vi "test_read-nmea-data2.vi"() -> ()   [LabVIEW 2019] (continued)
\t\n15:09:12.53\tF9P\t$GLGSV,2,2,08,77,01,327,,84,21,121,11,85,70,063,25,86,35,329,,1*72\n\t\n15:09:12.55\tF9P\t$GLGSV,2,1,08,69,13,031,18,70,73,042,,71,50,204,21,72,03,209,,3*79\n\t\n15:09:12.57\tF9P\t$GLGSV,2,2,08,77,01,327,,84,21,121,18,85,70,063,22,86,35,329,,3*7E\n\t\n15:09:12.59\tF9P\t$GAGSV,2,1,08,02,09,298,09,04,65,120,25,09,30,193,24,11,70,356,26,7*7E\n\t\n15:09:12.61\tF9P\t$GAGSV,2,2,08,12,41,101,23,19,27,046,13,25,10,250,,36,25,307,18,7*7F\n\t\n15:09:12.63\tF9P\t$GAGSV,2,1,08,02,09,298,,04,65,120,28,09,30,193,23,11,70,356,23,2*7D\n\t\n15:09:12.65\tF9P\t$GAGSV,2,2,08,12,41,101,18,19,27,046,,25,10,250,,36,25,307,23,2*78\n\t\n15:09:12.67\tF9P\t$GBGSV,1,1,03,11,51,130,24,14,86,148,24,33,59,218,31,1*40\n\t\n15:09:12.69\tF9P\t$GBGSV,1,1,04,08,,,22,11,51,130,22,14,86,148,26,33,59,218,,3*4B\n\t\n15:09:12.71\tF9P\t$GNGLL,3723.60695,N,12656.91212,E,060914.00,A,A*7B\n\t\n15:09:12.73\tF9P\t\t\n15:09:12.75\tF9P\t\t\n15:09:12.77\tF9P\t\t\n15:09:12.79\tF9P\t\t\n15:09:12.81\tF9P\t\t\n15:09:12.83\tF9P\t\t\n15:09:12.85\tF9P\t\t\n15:09:12.87\tF9P\t\t\n15:09:12.89\tF9P\t\t\n15:09:12.91\tF9P\t\t\n15:09:12.93\tF9P\t\t\n15:09:12.95\tF9P\t\t\n15:09:12.97\tF9P\t\t\n15:09:12.99\tF9P\t\t\n15:09:13.01\tF9P\t\t\n15:09:13.03\tF9P\t\t\n15:09:13.05\tF9P\t\t\n15:09:13.07\tF9P\t\t\n15:09:13.09\tF9P\t\t\n15:09:13.11\tF9P\t\t\n15:09:13.13\tF9P\t\t\n15:09:13.15\tF9P\t\t\n15:09:13.17\tF9P\t\t\n15:09:13.19\tF9P\t\t\n15:09:13.21\tF9P\t\t\n15:09:13.23\tF9P\t\t\n15:09:13.25\tF9P\t$GNRMC,060915.00,A,3723.60643,N,12656.91138,E,3.237,235.26,250720,,,A,V*00\n\t\n15:09:13.27\tF9P\t$GNVTG,235.26,T,,M,3.237,N,5.996,K,A*25\n\t\n15:09:13.30\tF9P\t$GNGGA,060915.00,3723.60643,N,12656.91138,E,1,12,0.73,59.2,M,18.5,M,,*7A\n\t\n15:09:13.32\tF9P\t$GNGSA,A,3,12,06,19,05,17,09,04,02,,,,,1.28,0.73,1.05,1*0B\n\t\n15:09:13.34\tF9P\t$GNGSA,A,3,85,71,84,,,,,,,,,,1.28,0.73,1.05,2*0E\n\t\n15:09:13.36\tF9P\t$GNGSA,A,3,36,19,11,04,09,12,,,,,,,1.28,0.73,1.05,3*0B\n\t\n15:09:13.38\tF9P\t$GNGSA,A,3,14,11,33,,,,,,,,,,1.28,0.73,1.05,4*0A\n\t\n15:09:13.40\tF9P\t$GPGSV,3,1,09,02,54,318,22,04,19,044,19,05,36,246,32,06,65,046,30,1*67\n\t\n15:09:13.42\tF9P\t$GPGSV,3,2,09,09,45,075,33,12,24,278,26,17,35,153,24,19,54,156,34,1*67\n\t\n15:09:13.44\tF9P\t$GPGSV,3,3,09,25,12,308,,1*52\n\t\n15:09:13.46\tF9P\t$GPGSV,3,1,09,02,54,318,,04,19,044,13,05,36,246,17,06,65,046,25,6*69\n\t\n15:09:13.48\tF9P\t$GPGSV,3,2,09,09,45,075,20,12,24,278,18,17,35,153,16,19,54,156,,6*69\n\t\n15:09:13.50\tF9P\t$GPGSV,3,3,09,25,12,308,,6*55\n\t\n15:09:13.52\tF9P\t$GLGSV,2,1,08,69,13,031,,70,73,042,,71,50,204,26,72,03,209,,1*75\n\t\n15:09:13.54\tF9P\t$GLGSV,2,2,08,77,01,327,,84,21,121,09,85,70,063,25,86,35,329,,1*7B\n\t\n15:09:13.56\tF9P\t$GLGSV,2,1,08,69,13,031,16,70,73,042,,71,50,204,22,72,03,209,,3*74\n\t\n15:09:13.58\tF9P\t$GLGSV,2,2,08,77,01,327,,84,21,121,17,85,70,063,21,86,35,329,,3*72\n\t\n15:09:13.60\tF9P\t$GAGSV,2,1,08,02,09,298,11,04,65,120,26,09,30,193,22,11,70,356,27,7*73\n\t\n15:09:13.62\tF9P\t$GAGSV,2,2,08,12,41,101,34,19,27,046,13,25,10,250,,36,25,307,17,7*76\n\t\n15:09:13.64\tF9P\t$GAGSV,2,1,08,02,09,298,,04,65,120,27,09,30,193,24,11,70,356,22,2*74\n\t\n15:09:13.66\tF9P\t$GAGSV,2,2,08,12,41,101,19,19,27,046,,25,10,250,,36,25,307,21,2*7B\n\t\n15:09:13.68\tF9P\t$GBGSV,1,1,03,11,51,130,24,14,86,148,26,33,59,218,31,1*42\n\t\n15:09:13.70\tF9P\t$GBGSV,1,1,04,08,,,23,11,51,130,23,14,86,148,25,33,59,218,,3*48\n\t\n15:09:13.72\tF9P\t$GNGLL,3723.60643,N,12656.91138,E,060915.00,A,A*7A\n\t\n15:09:13.74\tF9P\t\t\n15:09:13.76\tF9P\t\t\n15:09:13.78\tF9P\t\t\n15:09:13.80\tF9P\t\t\n15:09:13.82\tF9P\t\t\n15:09:13.84\tF9P\t\t\n15:09:13.86\tF9P\t\t\n15:09:13.88\tF9P\t\t\n15:09:13.90\tF9P\t\t\n15:09:13.92\tF9P\t\t\n15:09:13.94\tF9P\t\t\n15:09:13.96\tF9P\t\t\n15:09:13.98\tF9P\t\t\n15:09:14.00\tF9P\t\t\n15:09:14.02\tF9P\t\t\n15:09:14.04\tF9P\t\t\n15:09:14.06\tF9P\t\t\n15:09:14.08\tF9P\t\t\n15:09:14.10\tF9P\t\t\n15:09:14.12\tF9P\t\t\n15:09:14.14\tF9P\t\t\n15:09:14.16\tF9P\t\t\n15:09:14.18\tF9P\t\t\n15:09:14.20\tF9P\t\t\n15:09:14.22\tF9P\t\t\n15:09:14.24\tF9P\t\t\n15:09:14.26\tF9P\t$GNRMC,060916.00,A,3723.60597,N,12656.91090,E,1.962,233.87,250720,,,A,V*0E\n\t\n15:09:14.28\tF9P\t$GNVTG,233.87,T,,M,1.962,N,3.634,K,A*20\n\t\n15:09:14.30\tF9P\t$GNGGA,060916.00,3723.60597,N,12656.91090,E,1,12,0.73,59.3,M,18.5,M,,*71\n\t\n15:09:14.32\tF9P\t$GNGSA,A,3,12,06,19,05,17,09,04,02,,,,,1.28,0.73,1.05,1*0B\n\t\n15:09:14.34\tF9P\t$GNGSA,A,3,85,71,84,,,,,,,,,,1.28,0.73,1.05,2*0E\n\t\n15:09:14.36\tF9P\t$GNGSA,A,3,36,19,11,04,09,12,,,,,,,1.28,0.73,1.05,3*0B\n\t\n15:09:14.38\tF9P\t$GNGSA,A,3,14,11,33,,,,,,,,,,1.28,0.73,1.05,4*0A\n\t\n15:09:14.40\tF9P\t$GPGSV,3,1,09,02,54,318,23,04,19,044,19,05,36,246,26,06,65,046,33,1*60\n\t\n15:09:14.42\tF9P\t$GPGSV,3,2,09,09,45,075,29,12,24,278,31,17,34,153,25,19,54,156,31,1*6F\n\t\n15:09:14.44\tF9P\t$GPGSV,3,3,09,25,12,308,,1*52\n\t\n15:09:14.46\tF9P\t$GPGSV,3,1,09,02,54,318,,04,19,044,09,05,36,246,18,06,65,046,23,6*6B\n\t\n15:09:14.48\tF9P\t$GPGSV,3,2,09,09,45,075,22,12,24,278,18,17,34,153,16,19,54,156,,6*6A\n\t\n15:09:14.50\tF9P\t$GPGSV,3,3,09,25,12,308,,6*55\n\t\n15:09:14.52\tF9P\t$GLGSV,2,1,08,69,13,031,,70,73,042,,71,50,204,26,72,03,209,,1*75\n\t\n15:09:14.54\tF9P\t$GLGSV,2,2,08,77,01,327,,84,21,121,09,85,70,063,24,86,35,329,,1*7A\n\t\n15:09:14.56\tF9P\t$GLGSV,2,1,08,69,13,031,18,70,73,042,,71,50,204,21,72,03,209,,3*79\n\t\n15:09:14.58\tF9P\t$GLGSV,2,2,08,77,01,327,,84,21,121,17,85,70,063,21,86,35,329,,3*72\n\t\n15:09:14.60\tF9P\t$GAGSV,2,1,08,02,09,298,07,04,65,120,25,09,30,193,20,11,70,356,24,7*76\n\t\n15:09:14.62\tF9P\t$GAGSV,2,2,08,12,41,101,25,19,27,046,13,25,10,250,,36,25,307,19,7*78\n\t\n15:09:14.64\tF9P\t$GAGSV,2,1,08,02,09,298,,04,65,120,28,09,30,193,21,11,70,356,20,2*7C\n\t\n15:09:14.66\tF9P\t$GAGSV,2,2,08,12,41,101,19,19,27,046,,25,10,250,,36,25,307,27,2*7D\n\t\n15:09:14.68\tF9P\t$GBGSV,1,1,03,11,51,130,23,14,86,148,26,33,59,218,27,1*42\n\t\n15:09:14.70\tF9P\t$GBGSV,1,1,04,08,,,23,11,51,130,24,14,86,148,26,33,59,218,,3*4C\n\t\n15:09:14.72\tF9P\t$GNGLL,3723.60597,N,12656.91090,E,060916.00,A,A*70\n\t\n15:09:14.74\tF9P\t\t\n15:09:14.76\tF9P\t\t\n15:09:14.78\tF9P\t\t\n15:09:14.80\tF9P\t\t\n15:09:14.82\tF9P\t\t\n15:09:14.84\tF9P\t\t\n15:09:14.86\tF9P\t\t\n15:09:14.88\tF9P\t\t\n15:09:14.90\tF9P\t\t\n15:09:14.92\tF9P\t\t\n15:09:14.94\tF9P\t\t\n15:09:14.96\tF9P\t\t\n15:09:14.98\tF9P\t\t\n15:09:15.00\tF9P\t\t\n15:09:15.02\tF9P\t\t\n15:09:15.04\tF9P\t\t\n15:09:15.06\tF9P\t\t\n15:09:15.08\tF9P\t\t\n15:09:15.10\tF9P\t\t\n15:09:15.12\tF9P\t\t\n15:09:15.14\tF9P\t\t\n15:09:15.16\tF9P\t\t\n15:09:15.18\tF9P\t\t\n15:09:15.20\tF9P\t\t\n15:09:15.22\tF9P\t\t\n15:09:15.24\tF9P\t\t\n15:09:15.26\tF9P\t$GNRMC,060917.00,A,3723.60562,N,12656.91048,E,2.165,237.78,250720,,,A,V*08\n\t\n15:09:15.28\tF9P\t$GNVTG,237.78,T,,M,2.165,N,4.009,K,A*27\n\t\n15:09:15.30\tF9P\t$GNGGA,060917.00,3723.60562,N,12656.91048,E,1,12,0.67,59.3,M,18.5,M,,*7A\n\t\n15:09:15.32\tF9P\t$GNGSA,A,3,12,06,19,05,17,09,04,02,,,,,1.21,0.67,1.02,1*00\n\t\n15:09:15.34\tF9P\t$GNGSA,A,3,85,71,84,,,,,,,,,,1.21,0.67,1.02,2*05\n\t\n15:09:15.36\tF9P\t$GNGSA,A,3,36,19,11,04,09,12,,,,,,,1.21,0.67,1.02,3*00\n\t\n15:09:15.38\tF9P\t$GNGSA,A,3,14,11,33,,,,,,,,,,1.21,0.67,1.02,4*01\n\t\n15:09:15.40\tF9P\t$GPGSV,3,1,09,02,54,318,23,04,19,044,19,05,36,246,26,06,65,046,23,1*61\n\t\n15:09:15.42\tF9P\t$GPGSV,3,2,09,09,45,075,34,12,24,278,31,17,34,153,24,19,54,156,25,1*67\n\t\n15:09:15.44\tF9P\t$GPGSV,3,3,09,25,12,308,,1*52\n\t\n15:09:15.46\tF9P\t$GPGSV,3,1,09,02,54,318,,04,19,044,12,05,36,246,17,06,65,046,22,6*6F\n\t\n15:09:15.48\tF9P\t$GPGSV,3,2,09,09,45,075,22,12,24,278,18,17,34,153,15,19,54,156,,6*69\n\t\n15:09:15.50\tF9P\t$GPGSV,3,3,09,25,12,308,,6*55\n\t\n15:09:15.52\tF9P\t$GLGSV,2,1,08,69,13,031,,70,73,042,,71,50,204,31,72,03,209,,1*73\n\t\n15:09:15.54\tF9P\t$GLGSV,2,2,08,77,01,327,,84,21,121,10,85,70,063,31,86,35,329,,1*76\n\t\n15:09:15.56\tF9P\t$GLGSV,2,1,08,69,13,031,23,70,73,042,,71,50,204,22,72,03,209,,3*72\n\t\n15:09:15.58\tF9P\t$GLGSV,2,2,08,77,01,327,,84,21,121,18,85,70,063,20,86,35,329,,3*7C\n\t\n15:09:15.60\tF9P\t$GAGSV,2,1,08,02,09,298,11,04,65,120,25,09,30,193,22,11,70,356,23,7*74\n\t\n15:09:15.62\tF9P\t$GAGSV,2,2,08,12,41,101,24,19,27,046,13,25,10,250,,36,25,307,19,7*79\n\t\n15:09:15.64\tF9P\t$GAGSV,2,1,08,02,09,298,,04,65,120,32,09,30,193,20,11,70,356,20,2*76\n\t\n15:09:15.66\tF9P\t$GAGSV,2,2,08,12,41,101,19,19,27,046,,25,10,250,,36,25,307,28,2*72\n\t\n15:09:15.68\tF9P\t$GBGSV,1,1,03,11,51,130,23,14,86,148,26,33,59,218,27,1*42\n\t\n15:09:15.70\tF9P\t$GBGSV,1,1,04,08,,,22,11,51,130,21,14,86,148,26,33,59,218,,3*48\n\t\n15:09:15.72\tF9P\t$GNGLL,3723.60562,N,12656.91048,E,060917.00,A,A*7E\n\t\n15:09:15.74\tF9P\t\t\n15:09:15.76\tF9P\t\t\n15:09:15.78\tF9P\t\t\n15:09:15.80\tF9P\t\t\n15:09:15.82\tF9P\t\t\n15:09:15.84\tF9P\t\t\n15:09:15.86\tF9P\t\t\n15:09:15.88\tF9P\t\t\n15:09:15.90\tF9P\t\t\n15:09:15.92\tF9P\t\t\n15:09:15.94\tF9P\t\t\n15:09:15.96\tF9P\t\t\n15:09:15.98\tF9P\t\t\n15:09:16.00\tF9P\t\t\n15:09:16.02\tF9P\t\t\n15:09:16.04\tF9P\t\t\n15:09:16.06\tF9P\t\t\n15:09:16.08\tF9P\t\t\n15:09:16.10\tF9P\t\t\n15:09:16.12\tF9P\t\t\n15:09:16.14\tF9P\t\t\n15:09:16.16\tF9P\t\t\n15:09:16.18\tF9P\t\t\n15:09:16.20\tF9P\t\t\n15:09:16.22\tF9P\t\t\n15:09:16.24\tF9P\t\t\n15:09:16.26\tF9P\t$GNRMC,060918.00,A,3723.60529,N,12656.90999,E,2.086,239.76,250720,,,A,V*00\n\t\n15:09:16.28\tF9P\t$GNVTG,239.76,T,,M,2.086,N,3.863,K,A*28\n\t\n15:09:16.30\tF9P\t$GNGGA,060918.00,3723.60529,N,12656.90999,E,1,12,0.66,59.4,M,18.5,M,,*78\n\t\n15:09:16.32\tF9P\t$GNGSA,A,3,12,06,19,05,17,09,04,02,,,,,1.21,0.66,1.02,1*01\n\t\n15:09:16.34\tF9P\t$GNGSA,A,3,85,71,84,,,,,,,,,,1.21,0.66,1.02,2*04\n\t\n15:09:16.36\tF9P\t$GNGSA,A,3,36,19,11,04,09,12,,,,,,,1.21,0.66,1.02,3*01\n\t\n15:09:16.38\tF9P\t$GNGSA,A,3,14,11,33,,,,,,,,,,1.21,0.66,1.02,4*00\n\t\n15:09:16.40\tF9P\t$GPGSV,3,1,09,02,54,318,22,04,19,044,19,05,36,246,26,06,65,046,25,1*66\n\t\n15:09:16.42\tF9P\t$GPGSV,3,2,09,09,45,075,34,12,24,278,24,17,34,153,25,19,53,156,25,1*65\n\t\n15:09:16.44\tF9P\t$GPGSV,3,3,09,25,12,308,,1*52\n\t\n15:09:16.46\tF9P\t$GPGSV,3,1,09,02,54,318,,04,19,044,15,05,36,246,17,06,65,046,24,6*6E\n\t\n15:09:16.48\tF9P\t$GPGSV,3,2,09,09,45,075,22,12,24,278,17,17,34,153,13,19,53,156,,6*67\n\t\n15:09:16.50\tF9P\t$GPGSV,3,3,09,25,12,308,,6*55\n\t\n15:09:16.52\tF9P\t$GLGSV,2,1,08,69,13,031,,70,73,042,,71,50,204,34,72,03,209,,1*76\n\t\n15:09:16.54\tF9P\t$GLGSV,2,2,08,77,01,327,,84,21,121,12,85,70,063,24,86,35,329,,1*70\n\t\n15:09:16.56\tF9P\t$GLGSV,2,1,08,69,13,031,22,70,73,042,,71,50,204,24,72,03,209,,3*75\n\t\n15:09:16.58\tF9P\t$GLGSV,2,2,08,77,01,327,,84,21,121,17,85,70,063,20,86,35,329,,3*73\n\t\n15:09:16.60\tF9P\t$GAGSV,2,1,08,02,09,298,12,04,65,120,25,09,30,193,23,11,70,356,23,7*76\n\t\n15:09:16.62\tF9P\t$GAGSV,2,2,08,12,41,101,25,19,27,046,15,25,10,250,,36,25,307,19,7*7E\n\t\n15:09:16.64\tF9P\t$GAGSV,2,1,08,02,09,298,,04,65,120,27,09,30,193,20,11,70,356,22,2*70\n\t\n15:09:16.66\tF9P\t$GAGSV,2,2,08,12,41,101,17,19,27,046,,25,10,250,,36,25,307,27,2*73\n\t\n15:09:16.68\tF9P\t$GBGSV,1,1,03,11,51,130,22,14,86,148,25,33,59,218,26,1*41\n\t\n15:09:16.70\tF9P\t$GBGSV,1,1,04,08,,,21,11,51,130,22,14,86,148,26,33,59,218,,3*48\n\t\n15:09:16.72\tF9P\t$GNGLL,3723.60529,N,12656.90999,E,060918.00,A,A*7A\n\t\n15:09:16.74\tF9P\t\t\n15:09:16.76\tF9P\t\t\n15:09:16.78\tF9P\t\t\n15:09:16.80\tF9P\t\t\n15:09:16.82\tF9P\t\t\n15:09:16.84\tF9P\t\t\n15:09:16.86\tF9P\t\t\n15:09:16.88\tF9P\t\t\n15:09:16.90\tF9P\t\t\n15:09:16.92\tF9P\t\t\n15:09:16.94\tF9P\t\t\n15:09:16.96\tF9P\t\t\n15:09:16.98\tF9P\t\t\n15:09:17.00\tF9P\t\t\n15:09:17.02\tF9P\t\t\n15:09:17.04\tF9P\t\t\n15:09:17.06\tF9P\t\t\n15:09:17.08\tF9P\t\t\n15:09:17.10\tF9P\t\t\n15:09:17.12\tF9P\t\t\n15:09:17.14\tF9P\t\t\n15:09:17.16\tF9P\t\t\n15:09:17.18\tF9P\t\t\n15:09:17.20\tF9P\t\t\n15:09:17.22\tF9P\t\t\n15:09:17.24\tF9P\t$GNRMC,060919.00,A,3723.60505,N,12656.90947,E,1.416,,250720,,,A,\t\n15:09:17.26\tF9P\tV*15\n\t\n15:09:17.28\tF9P\t$GNVTG,,T,,M,1.416,N,2.622,K,A*3B\n\t\n15:09:17.30\tF9P\t$GNGGA,060919.00,3723.60505,N,12656.90947,E,1,12,0.76,59.2,M,18.5,M,,*73\n\t\n15:09:17.32\tF9P\t$GNGSA,A,3,12,06,19,05,17,09,04,02,,,,,1.33,0.76,1.09,1*08\n\t\n15:09:17.34\tF9P\t$GNGSA,A,3,85,71,84,,,,,,,,,,1.33,0.76,1.09,2*0D\n\t\n15:09:17.36\tF9P\t$GNGSA,A,3,36,19,11,04,09,12,,,,,,,1.33,0.76,1.09,3*08\n\t\n15:09:17.38\tF9P\t$GNGSA,A,3,14,11,33,,,,,,,,,,1.33,0.76,1.09,4*09\n\t\n15:09:17.40\tF9P\t$GPGSV,3,1,09,02,54,318,22,04,19,044,19,05,36,246,32,06,65,046,31,1*66\n\t\n15:09:17.42\tF9P\t$GPGSV,3,2,09,09,45,075,29,12,24,278,30,17,34,153,25,19,53,156,25,1*6C\n\t\n15:09:17.44\tF9P\t$GPGSV,3,3,09,25,12,308,,1*52\n\t\n15:09:17.46\tF9P\t$GPGSV,3,1,09,02,54,318,,04,19,044,15,05,36,246,18,06,65,046,25,6*60\n\t\n15:09:17.48\tF9P\t$GPGSV,3,2,09,09,45,075,19,12,24,278,18,17,34,153,13,19,53,156,,6*60\n\t\n15:09:17.50\tF9P\t$GPGSV,3,3,09,25,12,308,,6*55\n\t\n15:09:17.52\tF9P\t$GLGSV,2,1,08,69,13,031,,70,73,042,,71,50,204,30,72,03,209,,1*72\n\t\n15:09:17.54\tF9P\t$GLGSV,2,2,08,77,01,327,,84,21,121,13,85,70,063,30,86,35,329,,1*74\n\t\n15:09:17.56\tF9P\t$GLGSV,2,1,08,69,13,031,20,70,73,042,,71,50,204,23,72,03,209,,3*70\n\t\n15:09:17.58\tF9P\t$GLGSV,2,2,08,77,01,327,,84,21,121,16,85,70,063,21,86,35,329,,3*73\n\t\n15:09:17.60\tF9P\t$GAGSV,2,1,08,02,09,298,12,04,65,120,23,09,30,193,30,11,70,356,23,7*72\n\t\n15:09:17.62\tF9P\t$GAGSV,2,2,08,12,41,101,23,19,27,046,09,25,10,250,,36,25,307,18,7*74\n\t\n15:09:17.64\tF9P\t$GAGSV,2,1,08,02,09,298,,04,65,120,25,09,30,193,20,11,70,356,20,2*70\n\t\n15:09:17.66\tF9P\t$GAGSV,2,2,08,12,41,101,18,19,27,046,,25,10,250,,36,25,307,25,2*7E\n\t\n15:09:17.68\tF9P\t$GBGSV,1,1,03,11,51,130,22,14,86,148,25,33,59,218,26,1*41\n\t\n15:09:17.70\tF9P\t$GBGSV,1,1,04,08,,,23,11,51,130,22,14,86,148,25,33,59,218,,3*49\n\t\n15:09:17.72\tF9P\t$GNGLL,3723.60505,N,12656.90947,E,060919.00,A,A*76\n\t\n15:09:17.74\tF9P\t\t\n15:09:17.76\tF9P\t\t\n15:09:17.78\tF9P\t\t\n15:09:17.80\tF9P\t\t\n15:09:17.82\tF9P\t\t\n15:09:17.84\tF9P\t\t\n15:09:17.86\tF9P\t\t\n15:09:17.88\tF9P\t\t\n15:09:17.90\tF9P\t\t\n15:09:17.92\tF9P\t\t\n15:09:17.94\tF9P\t\t\n15:09:17.96\tF9P\t\t\n15:09:17.98\tF9P\t\t\n15:09:18.00\tF9P\t\t\n15:09:18.02\tF9P\t\t\n15:09:18.04\tF9P\t\t\n15:09:18.06\tF9P\t\t\n15:09:18.08\tF9P\t\t\n15:09:18.10\tF9P\t\t\n15:09:18.12\tF9P\t\t\n15:09:18.14\tF9P\t\t\n15:09:18.16\tF9P\t\t\n15:09:18.18\tF9P\t\t\n15:09:18.20\tF9P\t\t\n15:09:18.22\tF9P\t\t\n15:09:18.24\tF9P\t$GNRMC,060920.00,A,3723.60487,N,12656.90892,E,1.791,,250720,,,A,V*11\n\t\n15:09:18.26\tF9P\t$GNVTG,,T,,M,1.791,N,3.317,K,A*35\n\t\n15:09:18.28\tF9P\t$GNGGA,060920.00,3723.60487,N,12656.90892,E,1,12,0.73,59.7,M,18.5,M,,*7B\n\t\n15:09:18.30\tF9P\t$GNGSA,A,3,12,06,19,05,17,09,04,02,,,,,1.28,0.73,1.05,1*0B\n\t\n15:09:18.32\tF9P\t$GNGSA,A,3,85,71,84,,,,,,,,,,1.28,0.73,1.05,2*0E\n\t\n15:09:18.34\tF9P\t$GNGSA,A,3,36,19,11,04,09,12,,,,,,,1.28,0.73,1.05,3*0B\n\t\n15:09:18.36\tF9P\t$GNGSA,A,3,14,11,33,,,,,,,,,,1.28,0.73,1.05,4*0A\n\t\n15:09:18.38\tF9P\t$GPGSV,3,1,09,02,54,318,21,04,19,044,20,05,36,246,18,06,65,046,31,1*67\n\t\n15:09:18.40\tF9P\t$GPGSV,3,2,09,09,45,075,30,12,24,278,29,17,34,153,24,19,53,156,24,1*6C\n\t\n15:09:18.42\tF9P\t$GPGSV,3,3,09,25,12,308,,1*52\n\t\n15:09:18.44\tF9P\t$GPGSV,3,1,09,02,54,318,,04,19,044,16,05,36,246,18,06,65,046,24,6*62\n\t\n15:09:18.46\tF9P\t$GPGSV,3,2,09,09,45,075,18,12,24,278,18,17,34,153,11,19,53,156,,6*63\n\t\n15:09:18.48\tF9P\t$GPGSV,3,3,09,25,12,308,,6*55\n\t\n15:09:18.50\tF9P\t$GLGSV,2,1,08,69,13,031,,70,73,042,,71,50,204,29,72,03,209,,1*7A\n\t\n15:09:18.52\tF9P\t$GLGSV,2,2,08,77,01,327,,84,21,121,09,85,70,063,23,86,35,329,,1*7D\n\t\n15:09:18.54\tF9P\t$GLGSV,2,1,08,69,13,031,16,70,73,042,,71,50,204,22,72,03,209,,3*74\n\t\n15:09:18.56\tF9P\t$GLGSV,2,2,08,77,01,327,,84,21,121,16,85,70,063,21,86,35,329,,3*73\n\t\n15:09:18.58\tF9P\t$GAGSV,2,1,08,02,09,298,10,04,65,120,23,09,30,193,29,11,70,356,22,7*79\n\t\n15:09:18.60\tF9P\t$GAGSV,2,2,08,12,41,101,21,19,27,046,08,25,10,250,,36,25,307,17,7*78\n\t\n15:09:18.62\tF9P\t$GAGSV,2,1,08,02,09,298,,04,65,120,26,09,30,193,19,11,70,356,18,2*72\n\t\n15:09:18.64\tF9P\t$GAGSV,2,2,08,12,41,101,17,19,27,046,,25,10,250,,36,25,307,25,2*71\n\t\n15:09:18.66\tF9P\t$GBGSV,1,1,03,11,51,130,22,14,86,148,24,33,59,218,26,1*40\n\t\n15:09:18.68\tF9P\t$GBGSV,1,1,04,08,,,23,11,51,130,24,14,86,148,26,33,59,218,,3*4C\n\t\n15:09:18.70\tF9P\t$GNGLL,3723.60487,N,12656.90892,E,060920.00,A,A*7E\n\t\n15:09:18.72\tF9P\t\t\n15:09:18.74\tF9P\t\t\n15:09:18.76\tF9P\t\t\n15:09:18.78\tF9P\t\t\n15:09:18.80\tF9P\t\t\n15:09:18.82\tF9P\t\t\n15:09:18.84\tF9P\t\t\n15:09:18.86\tF9P\t\t\n15:09:18.88\tF9P\t\t\n15:09:18.90\tF9P\t\t\n15:09:18.92\tF9P\t\t\n15:09:18.94\tF9P\t\t\n15:09:18.96\tF9P\t\t\n15:09:18.98\tF9P\t\t\n15:09:19.00\tF9P\t\t\n15:09:19.02\tF9P\t\t\n15:09:19.04\tF9P\t\t\n15:09:19.06\tF9P\t\t\n15:09:19.08\tF9P\t\t\n15:09:19.10\tF9P\t\t\n15:09:19.12\tF9P\t\t\n15:09:19.14\tF9P\t\t\n15:09:19.16\tF9P\t\t\n15:09:19.18\tF9P\t\t\n15:09:19.20\tF9P\t\t\n15:09:19.22\tF9P\t\t\n15:09:19.24\tF9P\t$GNRMC,060921.00,A,3723.60462,N,12656.90824,E,2.232,238.97,250720,,,A,V*00\n\t\n15:09:19.26\tF9P\t$GNVTG,238.97,T,,M,2.232,N,4.134,K,A*27\n\t\n15:09:19.28\tF9P\t$GNGGA,060921.00,3723.60462,N,12656.90824,E,1,12,0.73,58.9,M,18.5,M,,*73\n\t\n15:09:19.30\tF9P\t$GNGSA,A,3,12,06,19,05,17,09,04,02,,,,,1.28,0.73,1.05,1*0B\n\t\n15:09:19.32\tF9P\t$GNGSA,A,3,85,71,84,,,,,,,,,,1.28,0.73,1.05,2*0E\n\t\n15:09:19.34\tF9P\t$GNGSA,A,3,36,19,11,04,09,12,,,,,,,1.28,0.73,1.05,3*0B\n\t\n15:09:19.36\tF9P\t$GNGSA,A,3,14,11,33,,,,,,,,,,1.28,0.73,1.05,4*0A\n\t\n15:09:19.38\tF9P\t$GPGSV,3,1,09,02,54,318,23,04,19,044,20,05,36,246,28,06,65,046,31,1*66\n\t\n15:09:19.40\tF9P\t$GPGSV,3,2,09,09,45,075,29,12,24,278,29,17,34,153,22,19,53,156,23,1*65\n\t\n15:09:19.42\tF9P\t$GPGSV,3,3,09,25,12,308,,1*52\n\t\n15:09:19.44\tF9P\t$GPGSV,3,1,09,02,54,318,,04,19,044,15,05,36,246,18,06,65,046,23,6*66\n\t\n15:09:19.46\tF9P\t$GPGSV,3,2,09,09,45,075,18,12,24,278,19,17,34,153,09,19,53,156,,6*6B\n\t\n15:09:19.48\tF9P\t$GPGSV,3,3,09,25,12,308,,6*55\n\t\n15:09:19.50\tF9P\t$GLGSV,2,1,08,69,13,031,,70,73,042,,71,50,204,29,72,03,209,,1*7A\n\t\n15:09:19.52\tF9P\t$GLGSV,2,2,08,77,01,327,,84,21,121,11,85,70,063,24,86,35,329,,1*73\n\t\n15:09:19.54\tF9P\t$GLGSV,2,1,08,69,13,031,15,70,73,042,,71,50,204,24,72,03,209,,3*71\n\t\n15:09:19.56\tF9P\t$GLGSV,2,2,08,77,01,327,,84,21,121,16,85,70,063,20,86,35,329,,3*72\n\t\n15:09:19.58\tF9P\t$GAGSV,2,1,08,02,09,298,10,04,65,120,22,09,30,193,20,11,70,356,21,7*72\n\t\n15:09:19.60\tF9P\t$GAGSV,2,2,08,12,41,101,20,19,27,046,11,25,10,250,,36,25,307,17,7*71\n\t\n15:09:19.62\tF9P\t$GAGSV,2,1,08,02,09,298,,04,65,120,32,09,30,193,18,11,70,356,19,2*77\n\t\n15:09:19.64\tF9P\t$GAGSV,2,2,08,12,41,101,18,19,27,046,,25,10,250,,36,25,307,22,2*79\n\t\n15:09:19.66\tF9P\t$GBGSV,1,1,03,11,51,130,22,14,86,148,25,33,59,218,26,1*41\n\t\n15:09:19.68\tF9P\t$GBGSV,1,1,04,08,,,23,11,51,130,21,14,86,148,27,33,59,218,,3*48\n\t\n15:09:19.70\tF9P\t$GNGLL,3723.60462,N,12656.90824,E,060921.00,A,A*79\n\t\n15:09:19.72\tF9P\t\t\n15:09:19.74\tF9P\t\t\n15:09:19.76\tF9P\t\t\n15:09:19.78\tF9P\t\t\n15:09:19.80\tF9P\t\t\n15:09:19.82\tF9P\t\t\n15:09:19.84\tF9P\t\t\n15:09:19.86\tF9P\t\t\n15:09:19.88\tF9P\t\t\n15:09:19.90\tF9P\t\t\n15:09:19.92\tF9P\t\t\n15:09:19.94\tF9P\t\t\n15:09:19.96\tF9P\t\t\n15:09:19.98\tF9P\t\t\n15:09:20.00\tF9P\t\t\n15:09:20.02\tF9P\t\t\n15:09:20.04\tF9P\t\t\n15:09:20.06\tF9P\t\t\n15:09:20.08\tF9P\t\t\n15:09:20.10\tF9P\t\t\n15:09:20.12\tF9P\t\t\n15:09:20.14\tF9P\t\t\n15:09:20.16\tF9P\t\t\n15:09:20.18\tF9P\t\t\n15:09:20.20\tF9P\t\t\n15:09:20.22\tF9P\t\t\n15:09:20.24\tF9P\t$GNRMC,060922.00,A,3723.60443,N,12656.90761,E,1.642,,250720,,,A,V*17\n\t\n15:09:20.26\tF9P\t$GNVTG,,T,,M,1.642,N,3.041,K,A*3A\n\t\n15:09:20.28\tF9P\t$GNGGA,060922.00,3723.60443,N,12656.90761,E,1,12,0.73,58.5,M,18.5,M,,*71\n\t\n15:09:20.30\tF9P\t$GNGSA,A,3,12,06,19,05,17,09,04,02,,,,,1.28,0.73,1.05,1*0B\n\t\n15:09:20.32\tF9P\t$GNGSA,A,3,85,71,84,,,,,,,,,,1.28,0.73,1.05,2*0E\n\t\n15:09:20.34\tF9P\t$GNGSA,A,3,36,19,11,04,09,12,,,,,,,1.28,0.73,1.05,3*0B\n\t\n15:09:20.36\tF9P\t$GNGSA,A,3,14,11,33,,,,,,,,,,1.28,0.73,
